vi "Format FP Properties Bullet List.vi"(8 "Error in":errorcluster caption="Error in (no error)", 11 "VI Info":T1) -> (0 "Error out":errorcluster, 3 "FP Properties Bullets":string)   [LabVIEW 2023, in "VIDoc Printer - Confluence.lvlib" / "VIDoc Printer - Confluence.lvclass"]
uses:
  VIDoc Printer - Confluence.lvclass
  Parsing/TypeDefs/Method Spec Cluster.ctl
  Parsing/TypeDefs/VI Type Extended Enum.ctl
  <vilib>/picture/picture.llb/imagedata.ctl
  Parsing/TypeDefs/Class Dispatch Type Enum.ctl
  Parsing/TypeDefs/Controls Info Cluster.ctl
  <vilib>/Utility/miscctls.llb/LVKeyTypeDef.ctl
  <vilib>/Utility/miscctls.llb/LVPointTypeDef.ctl
  Parsing/SubVIs/Structure Reporter/Tree Cluster.ctl
  VIDoc Printer - Confluence.lvclass/VIDoc Printer - Confluence.ctl
  Confluence Formatting/Confluence Formatting.lvlib
  Parsing/VIDoc Parsing.lvlib
  Parsing/SubVIs/Structure Reporter/Structure Reporter.lvlib
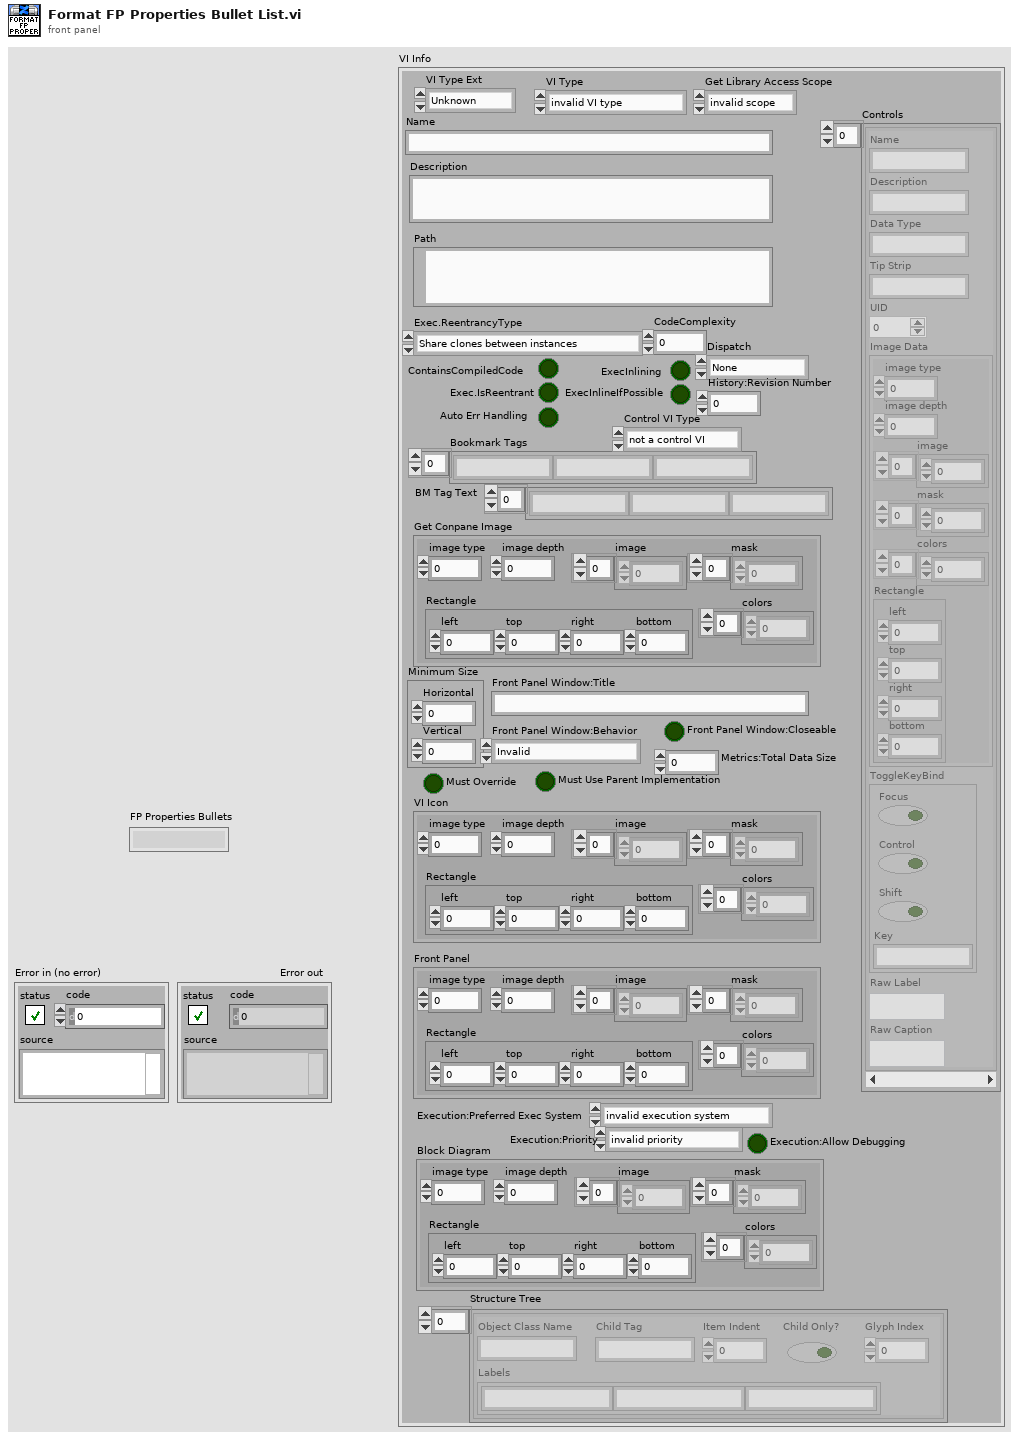
[diagram p1: front panel]
types:
  T1 = typedef "VIDoc Parsing.lvlib/Method Spec Cluster.ctl" = cluster{"VI Type Ext":T2, "Name":string, "Path":path, "Get Conpane Image":T3, "Description":string, "Get Library Access Scope":enum32{"invalid scope", "public", "private", "protected", "community"}, "Dispatch":T4, "ContainsCompiledCode":bool, "Exec.IsReentrant":bool, "Exec.ReentrancyType":enum16{"Share clones between instances", "Preallocate clone for each instance"}, "ExecInlining":bool, "ExecInlineIfPossible":bool, "Auto Err Handling":bool, "CodeComplexity":sgl, "Bookmark Tags":string[], "Control VI Type":enum32{"not a control VI", "control", "typedef", "strict typedef"}, "Controls":T5[], "VI Type":enum32{"invalid VI type", "Standard VI", "Control VI", "Global VI", "Polymorphic VI", "Configuration VI", "SubSystem", "Facade VI", "Method VI", "Statechart Diagram VI"}, "Minimum Size":T7, "Front Panel Window:Title":string, "Front Panel Window:Behavior":enum32{"Invalid", "Default", "Floating", "Floating/Auto-Hide", "Modal"}, "Front Panel Window:Closeable":bool, "Must Override":bool, "Must Use Parent Implementation":bool, "VI Icon":T3, "Front Panel":T3, "History:Revision Number":u32, "Metrics:Total Data Size":u32, "Execution:Allow Debugging":bool, "Execution:Preferred Exec System":enum32{"invalid execution system", "user interface", "standard", "instrument i/o", "data acquisition", "other 1", "other 2", "same as caller"}, "Execution:Priority":enum32{"invalid priority", "background priority", "normal priority", "above normal priority", "high priority", "time critical priority", "subroutine"}, "BM Tag Text":string[], "Block Diagram":T3, "Structure Tree":T8[]}
  T2 = typedef "VIDoc Parsing.lvlib/VI Type Extended Enum.ctl" = enum16{"Unknown", "Class Method", "Class Accessor Get", "Class Accessor Set", "Class Control", "Library Method", "Library Control", "VI", "Control"}
  T3 = typedef "imagedata.ctl" = cluster{"image type":i32, "image depth":i32, "image":u8[], "mask":u8[], "colors":u32[], "Rectangle":cluster{"left":i16, "top":i16, "right":i16, "bottom":i16}}
  T4 = typedef "VIDoc Parsing.lvlib/Class Dispatch Type Enum.ctl" = enum16{"None", "Static", "Dynamic"}
  T5 = typedef "VIDoc Parsing.lvlib/Controls Info Cluster.ctl" = cluster{"Name":string, "Description":string, "Data Type":string, "Tip Strip":string, "UID":i32, "Image Data":T3, "ToggleKeyBind":T6, "Raw Label":string, "Raw Caption":string}
  T6 = typedef "LVKeyTypeDef.ctl" = cluster{"Focus":bool, "Control":bool, "Shift":bool, "Key":string}
  T7 = typedef "LVPointTypeDef.ctl" = cluster{"Horizontal":i16, "Vertical":i16}
  T8 = typedef "VIDoc Parsing.lvlib/Structure Reporter.lvlib/Tree Cluster.ctl" = cluster{"Object Class Name":string, "Labels":string[], "Child Tag":string, "Item Indent":i32, "Child Only?":bool, "Glyph Index":i32}
  T9 = enum32{"Invalid", "Default", "Floating", "Floating/Auto-Hide", "Modal"}
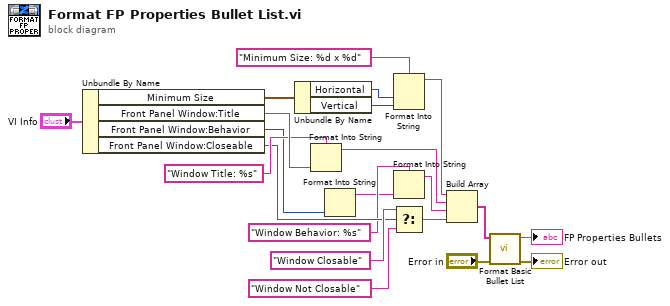
[diagram p0: block diagram]
diagram:
  n1 = Unbundle By Name("VI Info") -> ("Minimum Size"=w18:T7, "Front Panel Window:Title"=w13:string, "Front Panel Window:Behavior"=w7:T9, "Front Panel Window:Closeable"=w8:bool)
  n2 = Unbundle By Name(w18) -> ("Horizontal"=w17:i16, "Vertical"=w16:i16)
  n3 = Format Into String(format string="Window Title: %s", w13) -> (resulting string=w11:string)  [unwired: 2 in, 1 out]
  n4 = Format Into String(w7) -> (resulting string=w5:string)  [unwired: 3 in, 1 out]
  n5 = Format Into String(format string="Minimum Size: %d x %d", w17, w16) -> (resulting string=w15:string)  [unwired: 2 in, 1 out]
  n6 = Format Into String(format string="Window Behavior: %s", w5) -> (resulting string=w4:string)  [unwired: 2 in, 1 out]
  n7 = Select(t="Window Closable" ("format string"), s=w8, f="Window Not Closable" ("format string")) -> (s? t:f=w9:string)
  n8 = Build Array(w15, w11, w4, w9) -> (w1:string[])
  n9 = call "Format Basic Bullet List.vi"("Error in"="Error in", "String Array"=w1) -> ("Error out"=→"Error out":errorcluster, "Bullet List"=→"FP Properties Bullets":string)  [unwired: 8 in]
